vi "SENS_CORR_COLL_SESS_STEP.vi"(0 "VISA IN":refnum<visa-resource-name>, 5 "error in":errorcluster, 7 "Channel":i32, 9 "Session":i32) -> (14 "VISA Out":refnum<visa-resource-name>, 16 "Step":i32, 19 "error out":errorcluster)   [LabVIEW 2018, in "PNA-X.lvlib"]
doc: "SENS:CORR:COLL:SESS6:STEP?"
uses:
  PNA-X.lvlib
  Instance           1 32Saved   SENS_CORR_COLL_SESS_STEP .vi
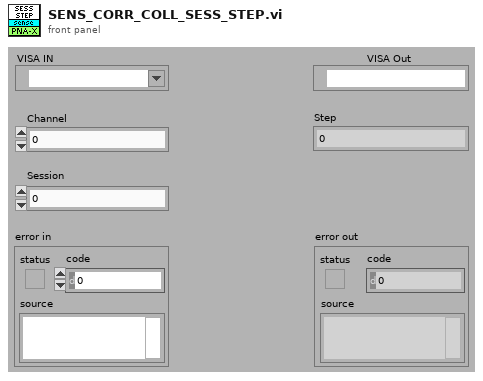
[diagram p1: front panel]
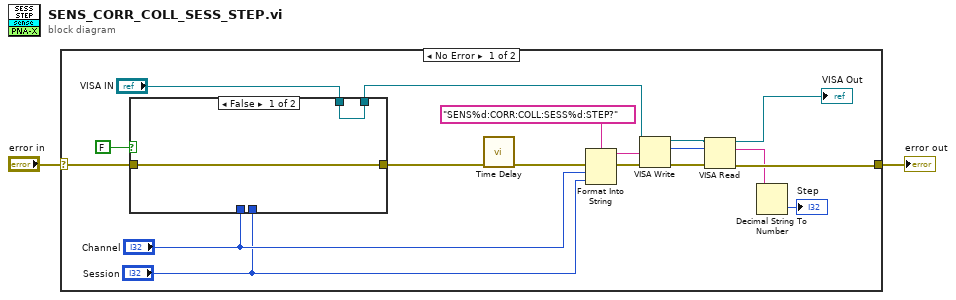
[diagram p0: block diagram]
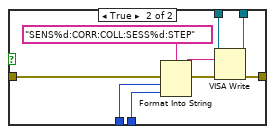
[diagram p2: hidden frame]
diagram:
  n1 = case shown="No Error" "error in" {
    selector: "error in" -> [w10 w32]
    tunnel: [w13 w32] -> w1
    frame No Error {
      n2 = case shown="False" FALSE {
        tunnel: w10 -> [w21 w29]
        tunnel: "VISA IN" -> [w22 w27]
        tunnel: "Channel" -> [_ w26]
        tunnel: "Session" -> [_ w25]
        tunnel: [w21 w24] -> w6
        tunnel: [w22 w23] -> w4
        frame False {
        }
        frame True {
          n3 = Format Into String(format string="SENS%d:CORR:COLL:SESS%d:STEP" ("Cmdline"), error in=w29, w26, w25) -> (resulting string=w31:string, error out=w30:errorcluster)  [unwired: 1 in]
          n4 = VISA Write(VISA resource name=w27, write buffer=w31, error in (no error)=w30) -> (VISA resource name out=w23:refnum<visa-resource-name>, error out=w24:errorcluster)  [unwired: 1 out]
        }
      }
      n5 = call "Time Delay"("error in (no error)"=w6) -> ("error out"=w5:errorcluster)  [unwired: 10 in]
      n6 = Format Into String(format string="SENS%d:CORR:COLL:SESS%d:STEP?" ("Cmdline"), error in=w5, "Channel", "Session") -> (resulting string=w19:string, error out=w20:errorcluster)  [unwired: 1 in]
      n7 = VISA Write(VISA resource name=w4, write buffer=w19, error in (no error)=w20) -> (VISA resource name out=w16:refnum<visa-resource-name>, return count=w15:u32, error out=w17:errorcluster)
      n8 = VISA Read(VISA resource name=w16, byte count=w15, error in (no error)=w17) -> (VISA resource name out=→"VISA Out":refnum<visa-resource-name>, read buffer=w12:string, error out=w13:errorcluster)  [unwired: 1 out]
      n9 = Decimal String To Number(string=w12) -> (number=→"Step":i32)  [unwired: 2 in, 1 out]
    }
    frame Error {
    }
  }
  "error out" <- w1
